vi "MGI File CheckValue.vi"(7 "CheckValue Type":T1, 8 "error in (no error)":errorcluster, 11 "File":path) -> (0 "error out":errorcluster, 2 "CheckSum":u32 format="0x%08x")   [LabVIEW 2016]
doc: "Calculate the Checkvalue for the specified file.\n\nFreeware from Moore Good Ideas, inc: www.MooreGoodIdeas.com. Do not remove this line."
uses:
  <userlib>/_MGI/File/Checksum/MGI CheckValue Method Enum.ctl
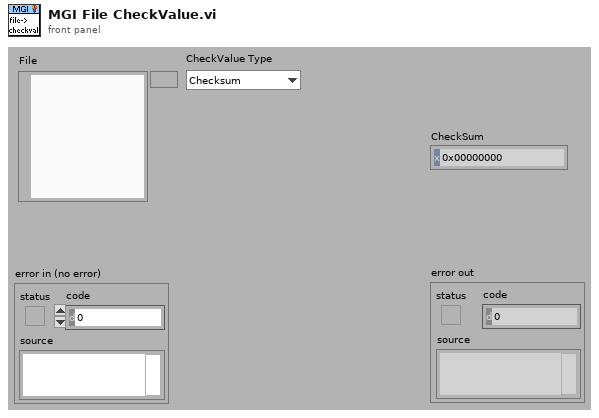
[diagram p1: front panel]
types:
  T1 = typedef "MGI CheckValue Method Enum.ctl" = enum16{"Checksum", "XOr"}
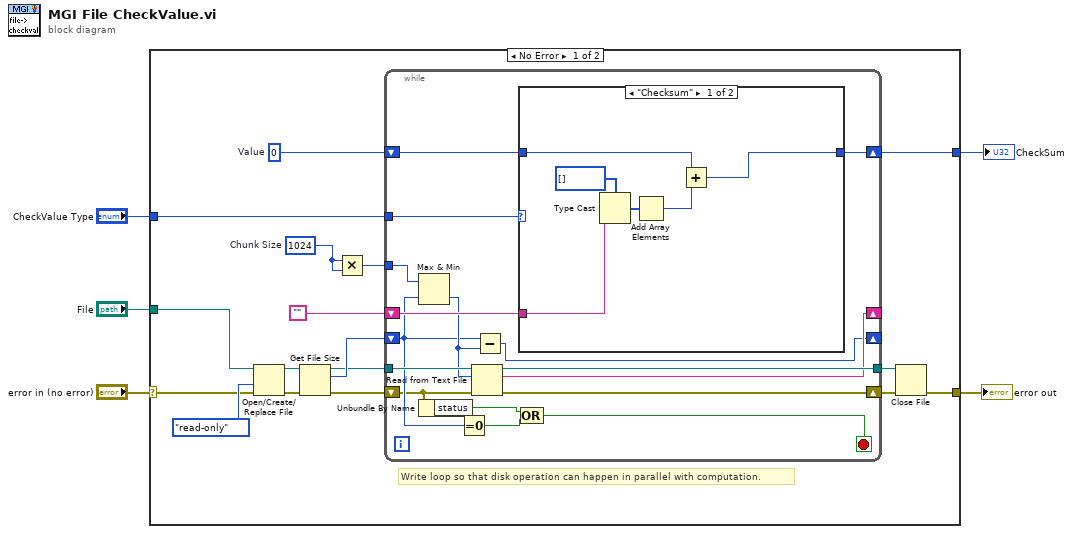
[diagram p0: block diagram]
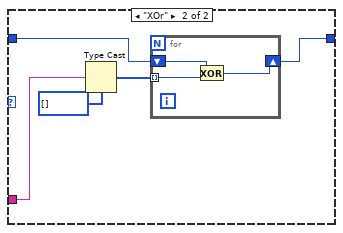
[diagram p2: hidden frame]
diagram:
  n1 = case shown="No Error" "error in (no error)" {
    selector: "error in (no error)" -> [w20 w53]
    tunnel: "CheckValue Type" -> [w11 _]
    tunnel: [w12 w53] -> w4
    tunnel: [w9 _] -> w3
    tunnel: "File" -> [w22 _]
    frame No Error {
      w7 = i64 1024  # Chunk Size
      w10 = u32 0  # Value
      # "Write loop so that disk operation can happen in parallel with computation."
      n2 = Open/Create/Replace File(file path (use dialog)=w22, error in=w20, access (0:read/write)=enum16{"read/write", "read-only", "write-only"}."read-only") -> (refnum out=w18:refnum<file>, error out=w19:errorcluster)  [unwired: 3 in, 1 out]
      n3 = Get File Size(file=w18, error in=w19) -> (refnum out=w15:refnum<file>, size (in bytes)=w16:i64, 0:w17:errorcluster)
      n4 = Multiply(x=w7, y=w7) -> (x*y=w6:i64)
      n5 = while {
        shift-right: [w28] -> w13
        shift-left: w17 -> [w26]
        shift-right: [w31] -> _
        shift-left: w16 -> [w27]
        tunnel: w6 -> [w38]
        tunnel: w15 -> [w37]
        tunnel: [w36] -> w14
        shift-right: [w35] -> _
        shift-left: "" -> [w34]
        tunnel: w11 -> [w33]
        shift-right: [w29] -> w9
        shift-left: w10 -> [w30]
        stop <- w23 stop-if-true
        n6 = Max & Min(x=w38, y=w27) -> (min(x,y)=w32:i64)  [unwired: 1 out]
        n7 = Unbundle By Name(w26) -> ("status"=w25:bool)
        n8 = Equal To 0?(x=w27) -> (x = 0?=w24:bool)
        n9 = Read from Text File(file (use dialog)=w37, count=w32, error in=w26) -> (refnum out=w36:refnum<file>, text=w35:string, error out=w28:errorcluster)  [unwired: 1 in, 1 out]
        n10 = Subtract(x=w27, y=w32) -> (x-y=w31:i64)
        n11 = case shown="\"Checksum\"" w33 {
          tunnel: w34 -> [w42 w48]
          tunnel: [w39 w46] -> w29
          tunnel: w30 -> [w41 w45]
          frame "Checksum" {
            n12 = Type Cast(type=u32[] [], x=w42) -> (*(type *) &x=w44:u32[])
            n13 = Add Array Elements(numeric array=w44) -> (sum=w40:u32)
            n14 = Add(x=w41, y=w40) -> (x+y=w39:u32)
          }
          frame "XOr" {
            n15 = Type Cast(type=u32[] [], x=w48) -> (*(type *) &x=w47:u32[])
            n16 = for {
              tunnel: w47 -> [w52] mode=indexing
              shift-right: [w51] -> w46
              shift-left: w45 -> [w50]
              n17 = Exclusive Or(1:w52, 2:w50) -> (0:w51:u32)
            }
          }
        }
        n18 = Compound Arithmetic op=OR(w25, w24) -> (w23:bool)
      }
      n19 = Close File(refnum=w14, error in=w13) -> (error out=w12:errorcluster)  [unwired: 1 out]
    }
    frame Error {
    }
  }
  "error out" <- w4
  "CheckSum" <- w3
